vi "FIR_5decimate_5cycles_finalstage.vi"(7 "reset":bool, 8 "valid in":bool, 10 "Q in":fxp<+/-,32,14>, 11 "I in":fxp<+/-,32,14>) -> (0 "valid out":bool, 2 "Q out":fxp<+/-,32,14>, 3 "I out":fxp<+/-,32,14>, 4 "ready for input":bool)   [LabVIEW 2025]
uses:
  <vilib>/rvi/IPIntegrationNode/IPINode_Typedef/niFpgaIPINodeSupportedFamilies.ctl
  <vilib>/rvi/FXPMathLib/FxpConvert/subVIs/nifxpmath_Convert_SimConfig.ctl
  <vilib>/fxp/LVFixedPointQuantizationPolicyTypeDef.ctl
  <vilib>/fxp/LVFixedPointOverflowPolicyTypeDef.ctl
  <vilib>/rvi/IPIntegrationNode/IPINode_Utilities/niFpgaIPINodeSimCore.vi
  <vilib>/rvi/FXPMathLib/FxpConvert/simVIs/DllFxpConvertTemp_sub.vi
  <vilib>/rvi/XilinxIP/XIPIN_XNode/niFpgaXIPIN.xnode
  Xilinx/FIR_5decimate_5cycles/xsim.dir/FIR_5decimate_5cycles_9B0F783A7DAD479FBAC8A1581EA5634C/xsimk_9B0F783A7DAD479FBAC8A1581EA5634C.dll
  <vilib>/rvi/IPIntegrationNode/IPINode_Xnode/niFpgaIPINode.xnode
  <vilib>/rvi/FXPMathLib/FxpInterpret/XNode/nifxpmath_Interpret.xnode
  <vilib>/rvi/FXPMathLib/FxpConvert/XNode/nifxpmath_Convert.xnode
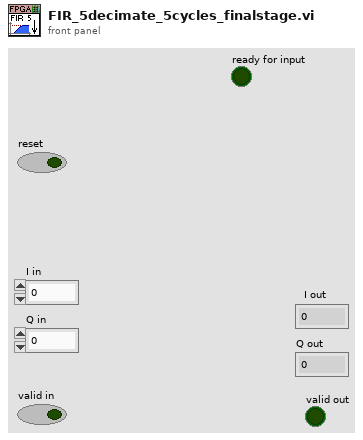
[diagram p1: front panel]
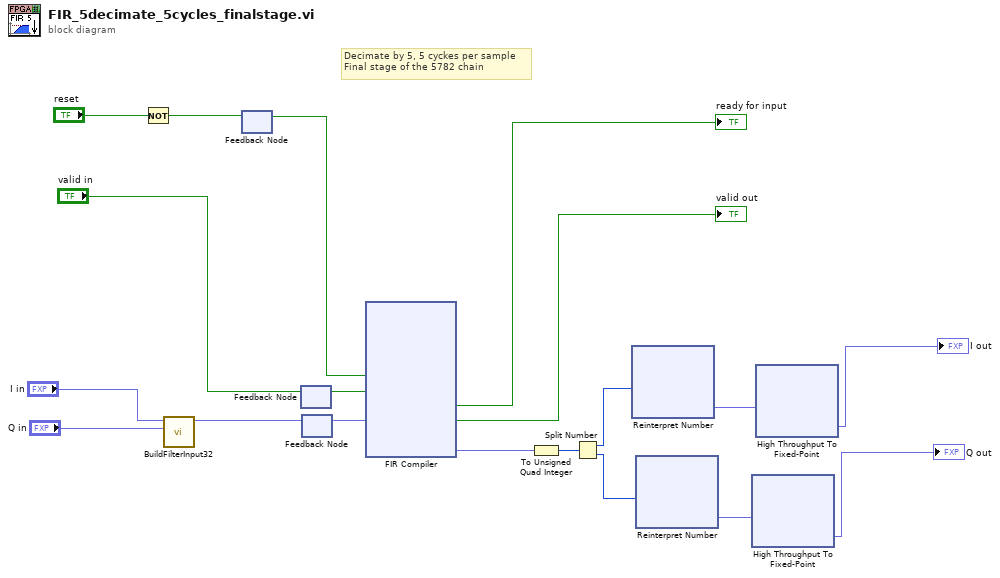
[diagram p0: block diagram]
diagram:
  # "Decimate by 5, 5 cyckes per sample\nFinal stage of the 5782 chain"
  n1 = Not(x="reset") -> (.not. x?=w2:bool)
  n2 = call "BuildFilterInput32.vi"("Q in"="Q in", "I in"="I in") -> ("Filter input"=w6:fxp<+,64,64>)  [unwired: 9 in]
  n3 = feedback #1() -> (w1:bool)  [unwired: 1 in]
  n4 = feedback-in #1(w2) -> ()
  n5 = feedback #2() -> (w3:bool)  [unwired: 1 in]
  n6 = feedback-in #2("valid in") -> ()
  n7 = feedback-in #3(w6) -> ()
  n8 = feedback #3() -> (w5:fxp<+,64,64>)  [unwired: 1 in]
  n9 = xnode ("FIR Compiler")("aresetn"=w1, "s_axis_data_tvalid"=w3, "s_axis_data_tdata"=w5) -> ("s_axis_data_tready"=→"ready for input":bool, "m_axis_data_tvalid"=→"valid out":bool, "m_axis_data_tdata"=w7:fxp<+,64,64>)  [unwired: 1 in]
  n10 = To Unsigned Quad Integer(1:w7) -> (0:w15:u64)
  n11 = Split Number(x=w15) -> (hi(x)=w16:u32, lo(x)=w12:u32)
  n12 = xnode "Reinterpret Number"("x"=w16) -> ("y"=w13:fxp<+/-,32,16>)
  n13 = xnode "Reinterpret Number"("x"=w12) -> ("y"=w14:fxp<+/-,32,16>)
  n14 = xnode "High Throughput To Fixed-Point"("x"=w14) -> ("y"=→"Q out":fxp<+/-,32,14>)
  n15 = xnode "High Throughput To Fixed-Point"("x"=w13) -> ("y"=→"I out":fxp<+/-,32,14>)
